vi "8-Tap 8-bit Camera with DRAM Modified (Host).vi"() -> ()   [LabVIEW 2013]
doc: "This is the host VI for the 10-Tap 8-Bit Camera with DRAM example. This example demonstrates how to acquire images from a 10-tap, 8-bit, extended configuration, Camera Link camera and display the images on the host. This example supports area scan and line scan cameras for both continuous and finite acquisitions.\n\nThis example also demonstrates the use of DRAM as a frame buffer for very high speed acquisitions. Data packing and flow-control are also employed to maximize use of the available DRAM and FIFOs in terms of both memory space and performance.\n\nAdditionally, the example demonstrates the serial server, which allows third-party camera configuration utilities to communicate with the camera using the Camera Link serial interface while this VI is running."
uses:
  <vilib>/userdefined/High Color/nirio_resource_hc.ctl
  <vilib>/rvi/interface/common/niFpgaWaitOnOcc.vi
  <vilib>/FPGAPlugInAG/PCIe-1473R/niLvFpga_Open_PCIe-1473R.vi
  <vilib>/rvi/interface/common/dynamic/niFpgaDynamicAddResources.vi
  <vilib>/FPGAPlugInAG/Dynamic/niLvFpga_Reset_Dynamic.vi
  <vilib>/Utility/error.llb/Error Cluster From Error Code.vi
  <vilib>/rvi/errors/niLvFpgaAdjustHostInterfaceError.vi
  <vilib>/FPGAPlugInAG/Dynamic/niLvFpga_Run_Dynamic.vi
  <vilib>/FPGAPlugInAG/Dynamic/niLvFpga_Close_Dynamic.vi
  <vilib>/rvi/interface/nirviOpenFPGA/nirviOpenFPGA.xnode
  FPGA Bitfiles/8-Tap8-bitCamera_FPGATarget_8-Tap8-bit.lvbitx
  <vilib>/rvi/interface/nirviMethod/nirviMethod.xnode
  <vilib>/rvi/interface/nirviReadWriteControl/nirviReadWriteControl.xnode
  <vilib>/rvi/interface/nirviCloseFPGA/nirviCloseFPGA.xnode
  NiFpgaLv.dll
  <vilib>/rvi/interface/Simulation/niFpgaSimulationCallBeginRW.vi
  <vilib>/rvi/errors/niLvFpgaMergeErrorWithErrorCode.vi
  <vilib>/FPGAPlugInAG/Dynamic/niLvFpga_ConfigureFifo_Dynamic.vi
  <vilib>/FPGAPlugInAG/Dynamic/niLvFpga_StartFifo_Dynamic.vi
  <vilib>/FPGAPlugInAG/Dynamic/niLvFpga_ReadFifo_Dynamic.vi
panel:
  in  "DMA Buffer Size\n(In Images)":u32=2200 caption="DMA Buffer Size"
  in  "Signal Mapping":T1(ring)
  out "Acq In Progress":bool
  in  "Line Scan":bool
  in  "Frames To Acquire":u32 caption="Frames To Acquire\n(0 = infinite)"
  in  "Cancel":bool
  out "Acq'd Frame Width":u32=1200
  in  "Stopped":bool=TRUE
  in  "RIO Device":T2="RIO0"
  out "DMA Write Timeout":bool
  in  "Start Serial Server":bool=TRUE
  out "Frames Acq'd":u32=593
  out "Acq'd Frame Height":u32=788
  out "Image":T3(plugin-control)
  in  "Acquire":bool
  in  "Stop":bool
  in  "Image Height":u32=788 max=65535
  in  "Image Width":u32=1200 max=65535 step=40
  out "Initialized":bool
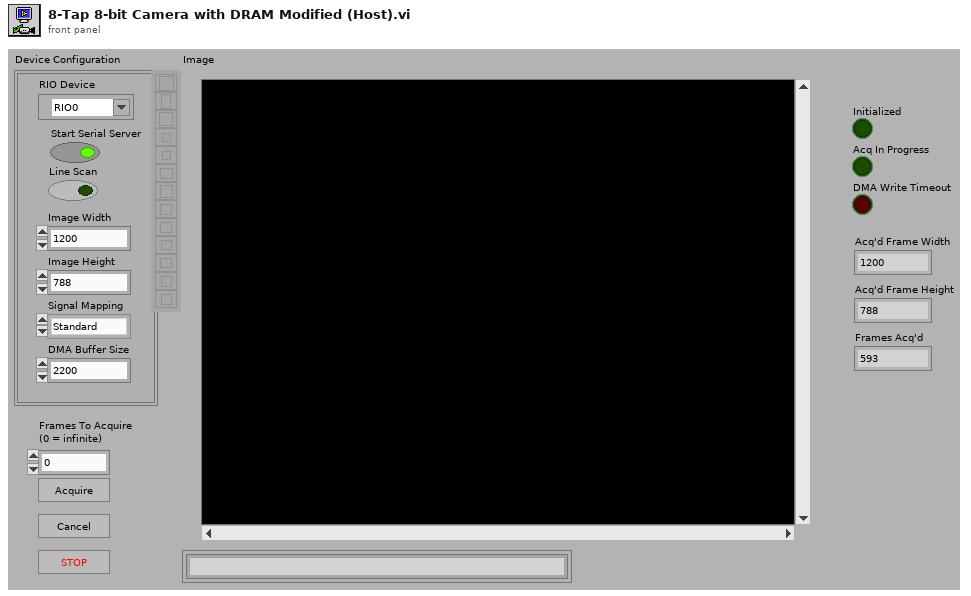
[diagram p1: front panel]
types:
  T1 = enum8{"Standard", "Basler 10-tap", "Vosskühler 10-tap"}
  T2 = typedef "nirio_resource_hc.ctl" = tag
  T3 = typedef "IMAQ Image.ctl" = refnum<image>
  T4 = typedef "Image Type" = u32
  T5 = enum16{"big-endian, network order", "native, host order", "little-endian"}
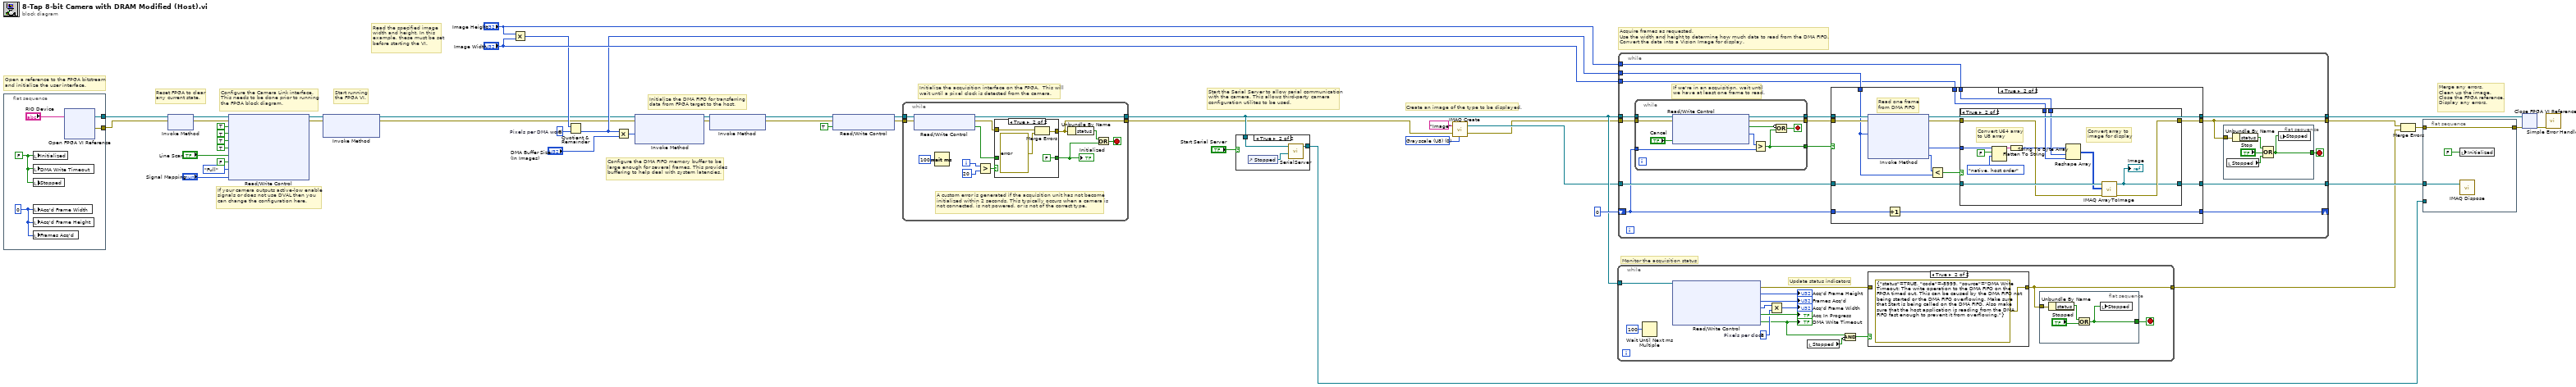
[diagram p0: block diagram]
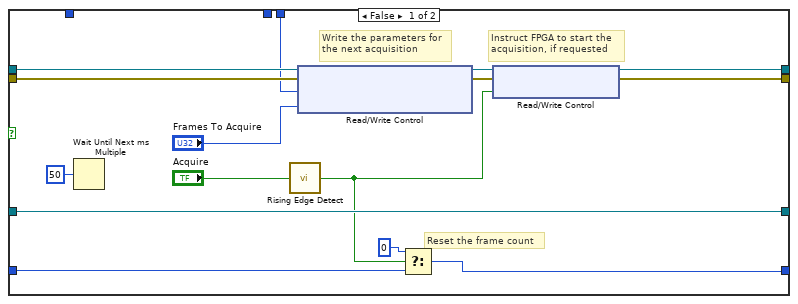
[diagram p4: hidden frame]
diagram:
  w5 = u32 8  # Pixels per DMA word
  w42 = T4 0 items=["Grayscale (U8)", "Grayscale (I16)", "Grayscale (SGL)", "Complex (CSG)", "RGB (U32)", "HSL (U32)", "RGB (U64)", "Grayscale (U16)"] ("Image Type")
  # "If your camera outputs active-low enable\nsignals or does not use DVAL then you \ncan change the configuration here."
  # "Configure the DMA FIFO memory buffer to be\nlarge enough for several frames. This provides\nbuffering to help deal with system latencies."
  # "Start running\nthe FPGA VI."
  # "Reset FPGA to clear\nany current state."
  # "Read the specified image\nwidth and height. In this\nexample, these must be set\nbefore starting the VI."
  # "Merge any errors.\nClean up the image.\nClose the FPGA reference.\nDisplay any errors."
  # "Acquire frames as requested.\nUse the width and height to determine how much data to read from the DMA FIFO.\nConvert the data into a Vision Image for display."
  # "Monitor the acquisition status"
  # "Start the Serial Server to allow serial communication\nwith the camera. This allows third-party camera\nconfiguration utilites to be used."
  # "Create an image of the type to be displayed."
  # "Initialize the acquisition interface on the FPGA.  This will\nwait until a pixel clock is detected from the camera."
  # "Initialize the DMA FIFO for transferring\ndata from FPGA target to the host."
  # "Configure the Camera Link interface.\nThis needs to be done prior to running\nthe FPGA block diagram."
  # "Open a reference to the FPGA bitstream\nand initialize the user interface."
  n1 = flat-sequence {
    tunnel: [w48] -> w33
    tunnel: [w47] -> w46
    frame #0 {
      w51 = u32 0 ("Num Lines Acq'd")
      w50 = FALSE ("stop")
      n2 = local write "Initialized"(w50) -> ()
      n3 = local write "DMA Write Timeout"(w50) -> ()
      n4 = local write "Stopped"(w50) -> ()
      n5 = local write "Acq'd Frame Width"(w51) -> ()
      n6 = local write "Acq'd Frame Height"(w51) -> ()
      n7 = local write "Frames Acq'd"(w51) -> ()
      n8 = xnode "Open FPGA VI Reference"("resource name"="RIO Device") -> ("FPGA VI Reference Out"=w48:refnum<k20>, "error out"=w47:errorcluster)  [unwired: 1 in]
    }
  }
  n9 = xnode "Invoke Method"("FPGA VI Reference In"=w33, "error in"=w46) -> ("FPGA VI Reference Out"=w22:refnum<k20>, "error out"=w25:errorcluster)
  n10 = xnode "Read/Write Control"("FPGA VI Reference In"=w22, "error in"=w25, "CL Config.FVAL Active High"=TRUE ("IO Module Config.CL FVAL Active High"), "CL Config.LVAL Active High"=TRUE ("IO Module Config.CL LVAL Active High"), "CL Config.DVAL Active High"=TRUE ("IO Module Config.CL DVAL Active High"), "CL Config.Spare Active High"=TRUE ("IO Module Config.CL Spare Active High"), "CL Config.Line Scan"="Line Scan", "Acq Control.Ignore DVAL"=FALSE ("CL Config.Line Scan"), "CL Config.Configuration"=enum8{"Base", "Medium", "Full"}."Full", "CL Config.Signal Mapping"="Signal Mapping") -> ("FPGA VI Reference Out"=w26:refnum<k20>, "error out"=w24:errorcluster)
  n11 = xnode "Invoke Method"("FPGA VI Reference In"=w26, "error in"=w24) -> ("FPGA VI Reference Out"=w2:refnum<k20>, "error out"=w1:errorcluster)  [unwired: 1 in]
  n12 = Multiply(x="Image Height", y="Image Width") -> (x*y=w4:u32)
  n13 = Quotient & Remainder(x=w4, y=w5) -> (floor(x/y)=w3:u32)  [unwired: 1 out]
  n14 = Multiply(x=w3, y="DMA Buffer Size\n(In Images)") -> (x*y=w16:u32)
  n15 = xnode "Invoke Method"("FPGA VI Reference In"=w2, "error in"=w1, "Requested Depth"=w16) -> ("FPGA VI Reference Out"=w32:refnum<k20>, "error out"=w31:errorcluster)  [unwired: 1 out]
  n16 = xnode "Invoke Method"("FPGA VI Reference In"=w32, "error in"=w31) -> ("FPGA VI Reference Out"=w17:refnum<k20>, "error out"=w30:errorcluster)
  n17 = xnode "Read/Write Control"("FPGA VI Reference In"=w17, "error in"=w30, "Acq Control.Initialize"=TRUE ("Arm Acquisition")) -> ("FPGA VI Reference Out"=w45:refnum<k20>, "error out"=w44:errorcluster)
  n18 = while {
    tunnel: w45 -> [w59]
    tunnel: w44 -> [w58]
    tunnel: [w57] -> w13
    tunnel: [w61] -> w12
    i -> [w53]
    stop <- w64 stop-if-true
    # "A custom error is generated if the acquisition unit has not become\ninitialized within 2 seconds. This typically occurs when a camera is\nnot connected, is not powered, or is not of the correct type."
    n19 = xnode "Read/Write Control"("FPGA VI Reference In"=w59, "error in"=w58) -> ("FPGA VI Reference Out"=w57:refnum<k20>, "error out"=w56:errorcluster, "Acq Status.Initialized"=w55:bool)
    n20 = Wait (ms)(milliseconds to wait=u32 100) -> ()  [unwired: 1 out]
    n21 = Greater?(x=w53, y=20) -> (0:w54:bool)
    n22 = case shown="True" w54 {
      tunnel: [w66 FALSE] -> w60
      tunnel: w55 -> [w66 _]
      tunnel: w56 -> [w65 w68]
      tunnel: [w65 w70] -> w61
      frame False {
      }
      frame True {
        n23 = Merge Errors(w68, errorcluster {"status"=TRUE, "code"=-8999, "source"="Acquisition Initialization: This error typically occurs when a camera is not properly connected, is not powered, or is not of the correct type."} ("error in")) -> (w70:errorcluster)
      }
    }
    "Initialized" <- w60
    n24 = Unbundle By Name(w61) -> ("status"=w63:bool)
    n25 = Or(x=w63, y=w60) -> (x .or. y?=w64:bool)
  }
  n26 = case shown="True" "Start Serial Server" {
    tunnel: [_ w71] -> w34
    tunnel: w13 -> [_ w72]
    frame False {
    }
    frame True {
      n27 = control-ref of="Stopped"() -> (w73:refnum<vi>)
      n28 = call "SerialServer.vi"("Stop Refnum"=w73, "FPGA VI Reference In"=w72) -> ("FPGA VI Reference Out"=w71:refnum<k20>)  [unwired: 5 in]
    }
  }
  n29 = call "IMAQ Create"("Image Name"="Image", "Image Type"=w42, "error in (no error)"=w12) -> ("New Image"=w9:T3, "error out"=w8:errorcluster)  [unwired: 2 in]
  n30 = while {
    tunnel: w13 -> [w84]
    tunnel: [w87] -> w27
    stop <- w86 stop-if-true
    w77 = u32 8  # Pixels per clock
    # "Update status indicators"
    n31 = Wait Until Next ms Multiple(millisecond multiple=u32 100) -> ()  [unwired: 1 out]
    n32 = xnode "Read/Write Control"("FPGA VI Reference In"=w84) -> ("error out"=w83:errorcluster, "Acq Status.Lines Per Frame"=→"Acq'd Frame Height":u32, "Acq Status.Frames Acq'd"=→"Frames Acq'd":u32, "Acq Status.Clocks Per Line"=w78:u32, "Acq Status.Acq In Progress"=→"Acq In Progress":bool, "Acq Status.DMA Write Timeout"=w75:bool)  [unwired: 1 in, 1 out]
    "DMA Write Timeout" <- w75
    n33 = Multiply(x=w78, y=w77) -> (x*y=→"Acq'd Frame Width":u32)
    n34 = local read "Stopped"() -> (w74:bool)
    n35 = Compound Arithmetic op=AND(w75, invert w74) -> (w76:bool)
    n36 = case shown="True" w76 {
      tunnel: w83 -> [w92 _]
      tunnel: [w92 errorcluster {"status"=TRUE, "code"=-8999, "source"="DMA Write Timeout: The write operation to the DMA FIFO on the FPGA timed out. This can be caused by the DMA FIFO not being started or the DMA FIFO overflowing. Make sure that Start is being called on the DMA FIFO. Also make sure that the host application is reading from the DMA FIFO fast enough to prevent it from overflowing."} ("error out")] -> w87
      frame False {
      }
      frame True {
      }
    }
    n37 = flat-sequence {
      tunnel: w87 -> [w91]
      tunnel: [w89] -> w86
      frame #0 {
        n38 = Unbundle By Name(w91) -> ("status"=w90:bool)
        n39 = Or(x=w90, y="Stopped") -> (x .or. y?=w89:bool)
        n40 = local write "Stopped"(w89) -> ()
      }
    }
  }
  n41 = while {
    tunnel: w13 -> [w100]
    tunnel: w8 -> [w99]
    tunnel: w3 -> [w108]
    tunnel: "Image Height" -> [w107]
    tunnel: "Image Width" -> [w106]
    tunnel: w9 -> [w105]
    tunnel: [w103] -> w28
    tunnel: [w104] -> w41
    tunnel: [w101] -> w36
    shift-right: [w95] -> _
    shift-left: u32 0 -> [w94]
    stop <- w102 stop-if-true
    # "If we're in an acquisition, wait until\nwe have at least one frame to read."
    n42 = while {
      tunnel: w100 -> [w115]
      tunnel: w99 -> [w114]
      tunnel: [w112] -> w98
      tunnel: [w113] -> w97
      tunnel: w94 -> [w118]
      tunnel: [w116] -> w96
      stop <- w117 stop-if-true
      n43 = xnode "Read/Write Control"("FPGA VI Reference In"=w115, "error in"=w114, "Acq Control.Cancel Acq"="Cancel") -> ("FPGA VI Reference Out"=w113:refnum<k20>, "error out"=w112:errorcluster, "Acq Status.Acq In Progress"=w111:bool, "Acq Status.Frames Acq'd"=w110:u32)
      n44 = Greater?(x=w110, y=w118) -> (0:w116:bool)
      n45 = Compound Arithmetic op=OR(invert w111, w116) -> (w117:bool)
    }
    n46 = case shown="True" w96 {
      tunnel: w97 -> [w134 w146]
      tunnel: w98 -> [w133 w145]
      tunnel: w108 -> [_ w139]
      tunnel: w107 -> [w127 w153]
      tunnel: w106 -> [_ w152]
      tunnel: w105 -> [w138 w151]
      tunnel: [w129 w149] -> w103
      tunnel: [w132 w148] -> w104
      tunnel: [w138 w147] -> w101
      tunnel: w94 -> [w135 w144]
      tunnel: [w137 w143] -> w95
      frame False {
        # "Reset the frame count"
        # "Instruct FPGA to start the\nacquisition, if requested"
        # "Write the parameters for\nthe next acquisition"
        n47 = Wait Until Next ms Multiple(millisecond multiple=u32 50) -> ()  [unwired: 1 out]
        n48 = call "Rising Edge Detect.vi"("Input"="Acquire") -> ("Pulse"=w124:bool)  [unwired: 4 in]
        n49 = xnode "Read/Write Control"("FPGA VI Reference In"=w134, "error in"=w133, "Acq Control.Line Scan Height"=w127, "Acq Control.Frames To Acq"="Frames To Acquire") -> ("FPGA VI Reference Out"=w131:refnum<k20>, "error out"=w130:errorcluster)
        n50 = Select(t=u32 0, s=w124, f=w135) -> (s? t:f=w137:u32)
        n51 = xnode "Read/Write Control"("FPGA VI Reference In"=w131, "error in"=w130, "Acq Control.Acquire"=w124) -> ("FPGA VI Reference Out"=w132:refnum<k20>, "error out"=w129:errorcluster)
      }
      frame True {
        # "Read one frame\nfrom DMA FIFO"
        n52 = xnode "Invoke Method"("FPGA VI Reference In"=w146, "error in"=w145, "Number of Elements"=w139) -> ("FPGA VI Reference Out"=w148:refnum<k20>, "error out"=w150:errorcluster, "Data"=w142:u64[], "Elements Remaining"=w140:u32)  [unwired: 1 in]
        n53 = Increment(x=w144) -> (x+1=w143:u32)
        n54 = Less?(x=w140, y=w139) -> (x < y?=w141:bool)
        n55 = case shown="True" w141 {
          tunnel: w153 -> [_ w167]
          tunnel: w152 -> [_ w166]
          tunnel: w151 -> [w155 w165]
          tunnel: w150 -> [w154 w164]
          tunnel: [w154 w163] -> w149
          tunnel: [w155 w162] -> w147
          tunnel: w142 -> [_ w159]
          frame False {
            # "Do not display the image if we're falling behind in the acquisition."
          }
          frame True {
            # "Convert U64 array\nto U8 array"
            # "Convert array to\nimage for display"
            n56 = Flatten To String(anything=w159, prepend array or string size? (T)=FALSE, byte order (0:big-endian, network order)=T5."native, host order") -> (data string=w157:string)  [unwired: 1 in, 2 out]
            n57 = String To Byte Array(string=w157) -> (unsigned byte array=w156:u8[])
            n58 = Reshape Array(w156, w167, w166) -> (w161:u8[][])
            n59 = call "IMAQ ArrayToImage"("error in (no error)"=w164, "Image Pixels (U8)"=w161, "Image"=w165) -> ("error out"=w163:errorcluster, "Image Out"=w162:T3)  [unwired: 7 in]
            "Image" <- w162
          }
        }
      }
    }
    n60 = flat-sequence {
      tunnel: w103 -> [w121]
      tunnel: [w120] -> w102
      frame #0 {
        n61 = local read "Stopped"() -> (w119:bool)
        n62 = Unbundle By Name(w121) -> ("status"=w122:bool)
        n63 = Compound Arithmetic op=OR(w122, "Stop", w119) -> (w120:bool)
        n64 = local write "Stopped"(w120) -> ()
      }
    }
  }
  n65 = Merge Errors(w28, w27) -> (w29:errorcluster)
  n66 = flat-sequence {
    tunnel: w29 -> [w169]
    tunnel: [w169] -> w38
    tunnel: w36 -> [w170]
    tunnel: w34 -> [_]
    frame #0 {
      n67 = local write "Initialized"(FALSE ("Module Enabled")) -> ()
      n68 = call "IMAQ Dispose"("Image"=w170) -> ()  [unwired: 5 in, 1 out]
    }
  }
  n69 = xnode "Close FPGA VI Reference"("FPGA VI Reference In"=w41, "error in"=w38) -> ("error out"=w35:errorcluster)
  n70 = call <vilib>:"Simple Error Handler.vi"("error in (no error)"=w35) -> ()  [unwired: 4 in, 5 out]
